vi "CurrentInput_FBL.vi"(8 "Mode":u16(ring) items=["Log w/ Exp Z", "Log w/ Lin Z"], 9 "Maximum (pA)":dbl=9000.0, 10 "Current (pA)":dbl format="%.1f", 11 "Setpoint (A)":dbl=100.0) -> (2 "Setpoint (pA)":dbl, 3 "Filtered Current (pA)":dbl format="%.1f", 7 "Current Maxed?":bool)   [LabVIEW 2017]
uses:
  <vilib>/Analysis/3filter.llb/Filter Passband Type.ctl
  <userlib>/HapticSTM/HapticSTM.lvlib
  <vilib>/ptbypt/NI_PtbyPt.lvlib
  <vilib>/Analysis/NI_AALBase.lvlib
panel:
  out "Filtered x":dbl format="%0.2f"
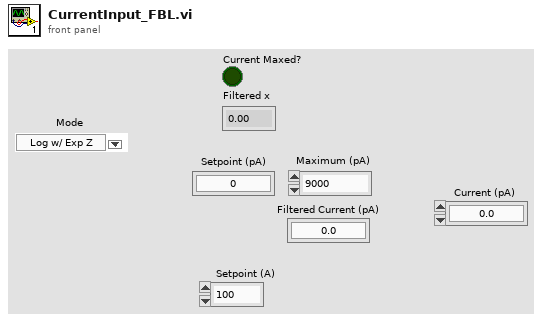
[diagram p1: front panel]
types:
  T1 = typedef "NI_AALBase.lvlib/Filter Passband Type.ctl" = enum32{"Lowpass", "Highpass", "Bandpass", "Bandstop"}
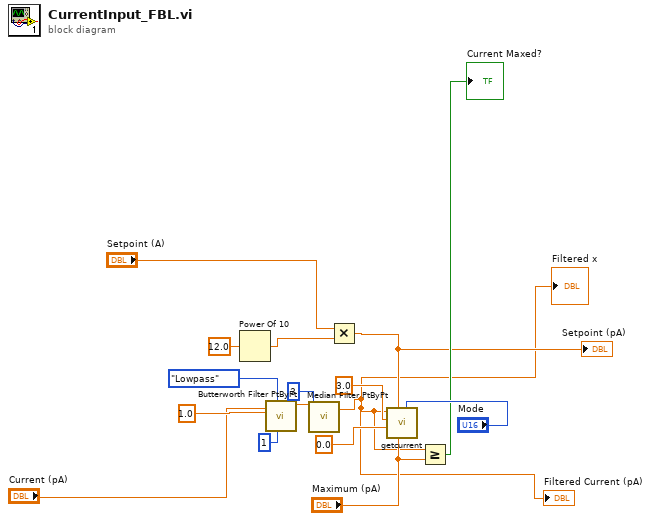
[diagram p0: block diagram]
diagram:
  n1 = Power Of 10(x=12.0) -> (10^x=w14:dbl)
  n2 = call <vilib>:"Butterworth Filter PtByPt.vi"("order"=1, "filter type"=Filter_Passband_Type."Lowpass", "sampling freq: fs"=1.0, "x"="Current (pA)") -> ("Filtered x"=w8:dbl)  [unwired: 5 in, 1 out]
  n3 = call <vilib>:"Median Filter PtByPt.vi"("rank"=3, "x"=w8) -> ("Filtered x"=w3:dbl)  [unwired: 2 in, 1 out]
  "Filtered Current (pA)" <- w3
  "Filtered x" <- w3
  n4 = Multiply(x="Setpoint (A)", y=w14) -> (x*y=w4:dbl)
  "Setpoint (pA)" <- w4
  n5 = call <userlib>:"getcurrent.vi"("forcemode"="Mode", "maxcurrentin"="Maximum (pA)", "setpoint"=w4, "minforcey"=0.0, "maxforcey"=3.0, "currentin"=w3) -> ()  [unwired: 6 in]
  n6 = Greater Or Equal?(x=w3, y="Maximum (pA)") -> (x >= y?=→"Current Maxed?":bool)
